vi "SLL DE AI Channel Type.vi"(8 "error in (no error)":errorcluster) -> (0 "error out":errorcluster, 1 "AI Channels Unit":T3(array[cluster]), 2 "AI Channel Type":T2[](array[typedef]), 3 "AI Channel Name":T1[](array[typedef]))   [LabVIEW 2013]
doc: "Copyright © 2005, Soliton Technologies.\nAll rights reserved."
uses:
  Controls/SLL DE DAQ Parameters LV2Global Options.ctl
  Controls/SLL DE List of AI Channel Type.ctl
  Controls/SLL DE List of Analog Inputs.ctl
  Controls/SLL DE Unit Info LV2Global Options.ctl
panel:
  in  "List of Analog Inputs":T1
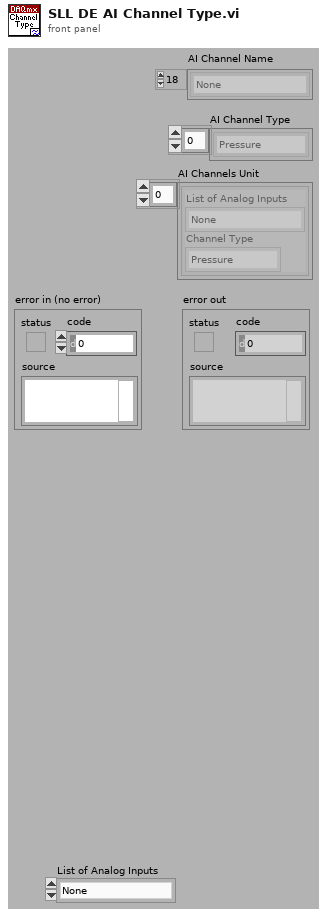
[diagram p1: front panel]
types:
  T1 = typedef "SLL DE List of Analog Inputs.ctl" = enum16{"None"}
  T2 = typedef "SLL DE List of AI Channel Type.ctl" = enum16{"Pressure", "Flow", "Temperature", "Time Scale", "Voltage", "Current", "Frequency", "Sound", "Speed", "Torque", "Distance", "Channel Type 1", "Channel Type 2", "Channel Type 3"}
  T3 = cluster{"List of Analog Inputs":T1, "Channel Type":T2}[]
  T4 = typedef "SLL DE Unit Info LV2Global Options.ctl" = enum16{"Update Channel Type", "Update Unit Info", "Get Unit Info", "Read"}
  T5 = typedef "SLL DE DAQ Parameters LV2Global Options.ctl" = enum16{"Read", "Write"}
  T6 = typedef "SLL DE DAQ Engine Parameters.ctl" = cluster{"Enable Engines":cluster{"AI Enable":bool, "AO Enable":bool, "DI Enable":bool, "DO Enable":bool}, "DAQ Control Type":cluster{"Analog Input":enum16{"Finite", "Continuous", "Driver"}, "Analog Output":enum16{"Finite", "Continuous", "Driver"}, "Digital Input":enum16{"Finite", "Continuous", "Driver"}, "Digital Output":enum16{"Finite", "Continuous", "Driver"}}, "DAQ Parameters":cluster{"AI Sampling Rate (Samples/Sec)":dbl, "MvgAVG Window Size (# of Points)":i32, "Enable Filter":bool, "Enable MvgAVG":bool, "Circular Buffer Size (Sec)":dbl, "AO Sampling Rate (Samples/Sec)":dbl, "Graph Update Rate (Samples/Sec)":dbl, "File Logging Rate (Samples/Sec)":i32}, "AO Safe Values":cluster{"Analog Outputs Name":T7, "Analog Outputs Safe Value":dbl}[], "DO Safe Values":cluster{"Digital Outputs Name":T8, "Digital Outputs Safe Value":bool}[], "DO Interconnected Lines":cluster{"First DO Line":string, "Second DO Line":string}[], "AI Channels Unit":cluster{"Channel Name":T1, "Channel Type":T2}[], "Units Information":cluster{"Channel Type":T2, "Unit Text":string, "Maximum":dbl, "Minmum":dbl, "Increments":dbl}[]}
  T7 = typedef "SLL DE List of Analog Outputs.ctl" = enum16{"None"}
  T8 = typedef "SLL DE List of Digital Outputs.ctl" = enum16{"STATION1_START TEST", "STATION1_STOP TEST", "STATION1_LIGHT1", "STATION1_LIGHT2", "STATION1_LIGHT3", "STATION1_SELECT_TEST", "STATION2_START TEST", "STATION2_STOP TEST", "STATION2_LIGHT1", "STATION2_LIGHT2", "STATION2_LIGHT3", "STATION2_SELECT_TEST", "STATION3_START TEST", "STATION3_STOP TEST", "STATION3_LIGHT1", "STATION3_LIGHT2", "STATION3_LIGHT3", "STATION3_SELECT_TEST", "STATION4_START TEST", "STATION4_STOP TEST", "STATION4_LIGHT1", "STATION4_LIGHT2", "STATION4_LIGHT3", "STATION4_SELECT_TEST"}
  T9 = cluster{"List of Analog Inputs":T1, "Channel Type":T2}
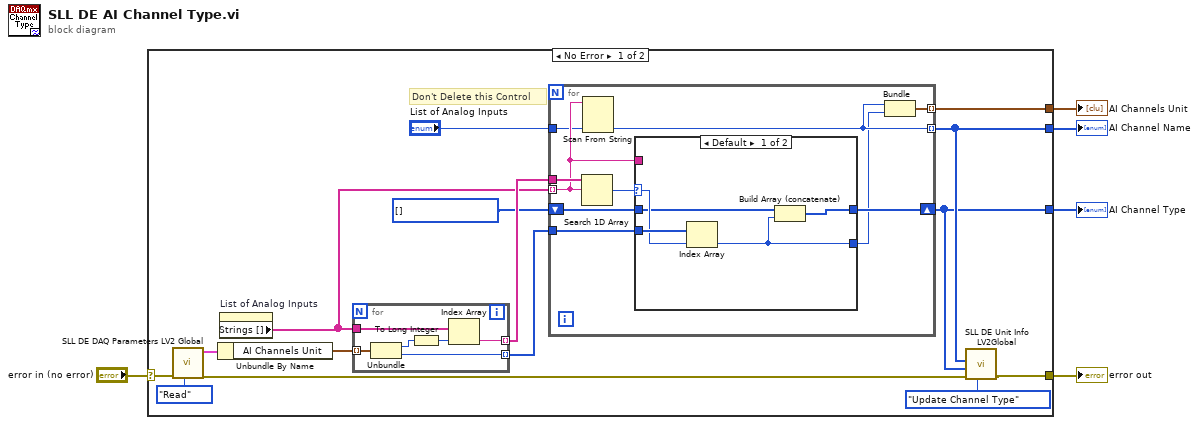
[diagram p0: block diagram]
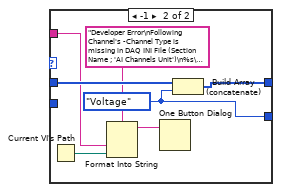
[diagram p2: hidden frame]
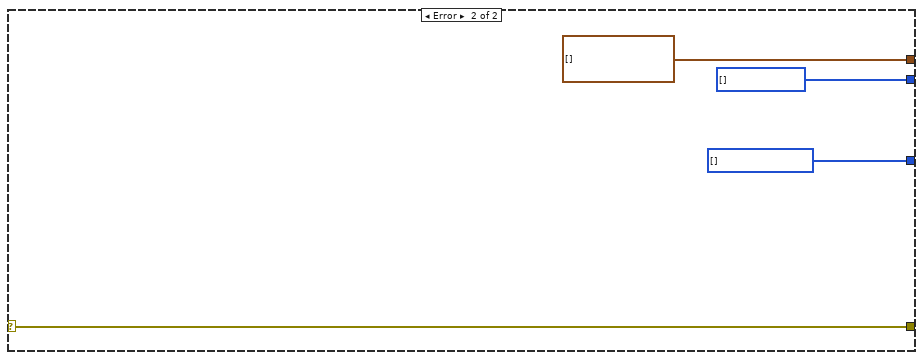
[diagram p3: hidden frame]
diagram:
  n1 = case shown="No Error" "error in (no error)" {
    selector: "error in (no error)" -> [w16 w52]
    tunnel: [w8 w52] -> w4
    tunnel: [w6 w51] -> w2
    tunnel: [w7 w50] -> w3
    tunnel: [w11 T3 []] -> w1
    frame No Error {
      w12 = T2[] [] items=["Pressure", "Flow", "Temperature", "Time Scale", "Voltage", "Current", "Frequency", "Sound", "Speed", "Torque", "Distance", "Channel Type 1", "Channel Type 2", "Channel Type 3"]
      # "Don't Delete this Control"
      n2 = call "SLL DE DAQ Parameters LV2 Global.vi"("Option"=SLL_DE_DAQ_Parameters_LV2Global_Options."Read", "Error in (no error)"=w16) -> ("Error out"=w9:errorcluster, "Global Info"=w18:T6)  [unwired: 8 in]
      n3 = Unbundle By Name(w18) -> ("AI Channels Unit"=w19:cluster{"Channel Name":T1, "Channel Type":T2}[])
      n4 = property on="List of Analog Inputs" class="Enum (strict)"() -> ("Strings []"=w14:string[])  [unwired: 2 in, 2 out]
      n5 = for {
        tunnel: w19 -> [w26] mode=indexing
        tunnel: w14 -> [w23]
        tunnel: [w22] -> w15 mode=indexing
        tunnel: [w21] -> w13 mode=indexing
        n6 = Unbundle(w26) -> ("Channel Name"=w25:T1, "Channel Type"=w21:T2)
        n7 = To Long Integer(number=w25) -> (32bit integer=w24:i32)
        n8 = Index Array(array=w23, index=w24) -> (element=w22:string)
      }
      n9 = for {
        tunnel: w15 -> [w36]
        tunnel: w14 -> [w31] mode=indexing
        tunnel: w13 -> [w34]
        shift-right: [w33] -> w6
        shift-left: w12 -> [w32]
        tunnel: "List of Analog Inputs" -> [w30]
        tunnel: [w29] -> w7 mode=indexing
        tunnel: [w27] -> w11 mode=indexing
        n10 = Search 1D Array(1D array=w36, element=w31) -> (index of element=w35:i32)  [unwired: 1 in]
        n11 = Scan From String(input string=w31, default 1=w30) -> (output 1=w29:T1)  [unwired: 3 in, 3 out]
        n12 = case shown="Default" w35 {
          selector: w35 -> [w40 _]
          tunnel: w34 -> [w41 _]
          tunnel: [w39 w47] -> w33
          tunnel: w32 -> [w38 w48]
          tunnel: w31 -> [_ w44]
          tunnel: [w37 w42] -> w28
          frame Default {
            n13 = Index Array(array=w41, index=w40) -> (element=w37:T2)
            n14 = Build Array (concatenate)(w38, w37) -> (w39:T2[])
          }
          frame -1 {
            w42 = SLL_DE_List_of_AI_Channel_Type."Voltage" ("Channel Type")
            n15 = Current VI's Path() -> (path=w46:path)
            n16 = Format Into String(format string="Developer Error\nFollowing Channel's -Channel Type is missing in DAQ INI File (Section Name ; 'AI Channels Unit')\n%s\n%s" ("message"), w44, w46) -> (resulting string=w45:string)  [unwired: 2 in, 1 out]
            n17 = One Button Dialog(message=w45) -> ()  [unwired: 1 in, 1 out]
            n18 = Build Array (concatenate)(w48, w42) -> (w47:T2[])
          }
        }
        n19 = Bundle("List of Analog Inputs"=w29, "Channel Type"=w28) -> (w27:T9)  [unwired: 1 in]
      }
      n20 = call "SLL DE Unit Info LV2Global.vi"("Option"=SLL_DE_Unit_Info_LV2Global_Options."Update Channel Type", "Error in (no error)"=w9, "AI Channel Type"=w6, "AI Channel Names"=w7) -> ("Error out"=w8:errorcluster)  [unwired: 5 in, 2 out]
    }
    frame Error {
      w51 = T2[] [] items=["Pressure", "Flow", "Temperature", "Time Scale", "Voltage", "Current", "Frequency", "Sound", "Speed", "Torque", "Distance", "Channel Type 1", "Channel Type 2", "Channel Type 3"] ("DO Safe Values")
      w50 = T1[] [] items=["None"]
    }
  }
  "error out" <- w4
  "AI Channel Name" <- w3
  "AI Channel Type" <- w2
  "AI Channels Unit" <- w1
